vi "SX.vi"(8 "error in (no error)":errorcluster, 9 "Valor":string, 10 "Puerto":u8, 11 "Serial Devices in":refnum<class "Serial Devices.lvclass">) -> (0 "error out":errorcluster, 3 "Serial Devices out":refnum<class "Serial Devices.lvclass">)   [LabVIEW 2019, in "Serial Devices.lvlib" / "Serial Devices.lvclass"]
uses:
  Serial Devices.lvclass
  C:/Program Files (x86)/National Instruments/LabVIEW 2019/vi.lib/ActorFramework/Actor/Actor.lvclass
  Serial Devices.lvclass/Serial Devices.ctl
  <vilib>/ActorFramework/Actor/Actor.lvclass/Actor.ctl
  <vilib>/ActorFramework/Message Enqueuer/Message Enqueuer.lvclass/Message Enqueuer.ctl
  NXP/NXP.lvclass
  TI/CYPRESS.lvclass
  SIMULATED/SIMULATED.lvclass
  <vilib>/ActorFramework/Message Enqueuer/Init from Existing Queue.vi
  <vilib>/ActorFramework/Message Enqueuer/Message Enqueuer.lvclass
  <vilib>/ActorFramework/Actor/Actor.lvclass
  Serial Devices.lvlib
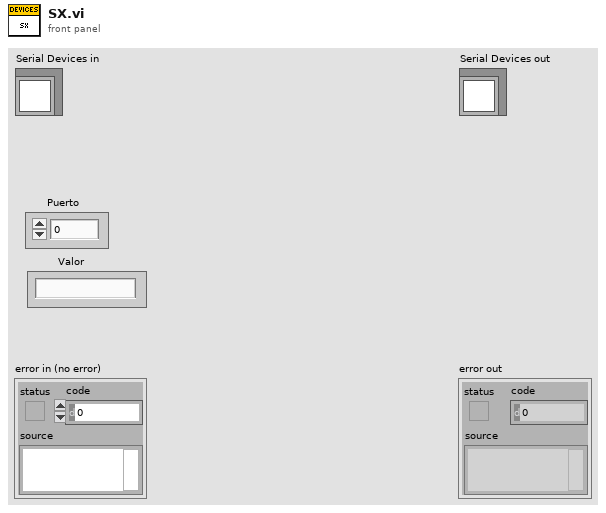
[diagram p1: front panel]
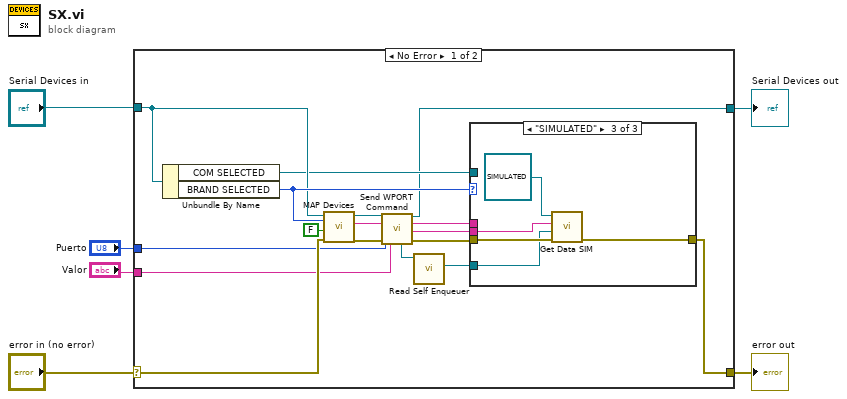
[diagram p0: block diagram]
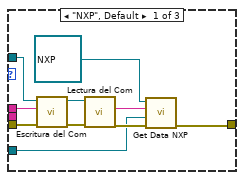
[diagram p2: hidden frame]
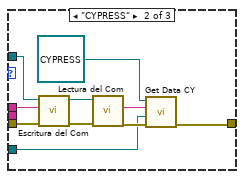
[diagram p3: hidden frame]
diagram:
  n1 = case shown="No Error" "error in (no error)" {
    selector: "error in (no error)" -> [w21 w49]
    tunnel: [w18 w49] -> w5
    tunnel: [w15 w48] -> w3
    tunnel: "Serial Devices in" -> [w17 w48]
    tunnel: "Puerto" -> [w10 _]
    tunnel: "Valor" -> [w7 _]
    frame No Error {
      n2 = Unbundle By Name(w17) -> ("COM SELECTED"=w16:refnum<visa-resource-name>, "BRAND SELECTED"=w20:enum16{"NXP", "CYPRESS", "SIMULATED"})
      n3 = call "MAP Devices.vi"("error in (no error)"=w21, "CREAR"=FALSE, "BRAND SELECTED"=w20, "Serial Devices in"=w17) -> ("error out"=w9:errorcluster, "VALOR"=w11:string, "Serial Devices out"=w8:refnum<class "Serial Devices.lvclass">)  [unwired: 5 in]
      n4 = call-dynamic "Send WPORT Command.vi"("Serial Devices in"=w8, "Device"=w11, "Puerto"=w10, "Valor"=w7, "error in"=w9) -> ("Serial Devices out"=w15:refnum<class "Serial Devices.lvclass">, "Command"=w14:string, "Expected"=w13:string, "error out"=w12:errorcluster)  [unwired: 7 in]
      n5 = call <vilib>:"Read Self Enqueuer.vi"("Actor"=w8) -> ("Self Enqueuer"=w19:refnum<class "Message Enqueuer.lvclass">)  [unwired: 10 in]
      n6 = case shown="\"SIMULATED\"" w20 {
        tunnel: w12 -> [w32 w42 w46]
        tunnel: w13 -> [_ _ w45]
        tunnel: w19 -> [w24 w34 w44]
        tunnel: [w23 w33 w43] -> w18
        tunnel: w16 -> [w30 w41 _]
        tunnel: w14 -> [w31 w40 _]
        frame "NXP", Default {
          n7 = call "Escritura del Com.vi"("error in (no error)"=w32, "write buffer"=w31, "VISA Refnum in"=w30) -> ("error out"=w28:errorcluster, "VISA resource name out"=w29:refnum<visa-resource-name>)  [unwired: 7 in]
          n8 = call "Lectura del Com.vi"("error in (no error)"=w28, "VISA Refnum in"=w29) -> ("error out"=w25:errorcluster, "Serial Response"=w26:string)  [unwired: 7 in, 1 out]
          n9 = call "Get Data NXP.vi"("error in"=w25, "Data Enqueuer"=w24, "Data"=w26, "NXP in"=refnum<class "NXP.lvclass"> refnum ("NXP.lvclass")) -> ("error out"=w23:errorcluster)  [unwired: 6 in, 1 out]
        }
        frame "CYPRESS" {
          n10 = call "Escritura del Com.vi"("error in (no error)"=w42, "write buffer"=w40, "VISA Refnum in"=w41) -> ("error out"=w39:errorcluster, "VISA resource name out"=w38:refnum<visa-resource-name>)  [unwired: 7 in]
          n11 = call "Lectura del Com.vi"("error in (no error)"=w39, "VISA Refnum in"=w38) -> ("error out"=w35:errorcluster, "Serial Response"=w36:string)  [unwired: 7 in, 1 out]
          n12 = call "Get Data CY.vi"("error in"=w35, "Data Enqueuer"=w34, "Data"=w36, "CYPRESS in"=refnum<class "CYPRESS.lvclass"> refnum ("CYPRESS.lvclass")) -> ("error out"=w33:errorcluster)  [unwired: 6 in, 1 out]
        }
        frame "SIMULATED" {
          n13 = call "Get Data SIM.vi"("error in"=w46, "Data Enqueuer"=w44, "Data"=w45, "SIMULATED in"=refnum<class "SIMULATED.lvclass"> refnum ("SIMULATED.lvclass")) -> ("error out"=w43:errorcluster)  [unwired: 6 in, 1 out]
        }
      }
    }
    frame Error {
    }
  }
  "error out" <- w5
  "Serial Devices out" <- w3
